vi "scrollToZoom.vi"(8 "stop":refnum<vi>, 9 "Don't need to press Ctrl To ZoomIn/ZoomOut":bool, 10 "ROI數量":i32=1, 11 "VI in":refnum<vi>) -> ()   [LabVIEW 2015]
panel:
  in  "stop":bool
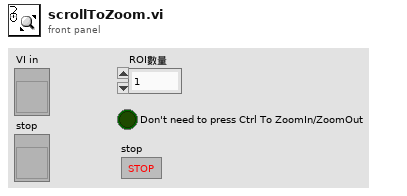
[diagram p1: front panel]
types:
  T1 = cluster{"ImageDataArray":cluster{"ImageName":string, "ImageZoom":dbl}, refnum<vi>}[]
  T2 = cluster{cluster{"Label.Text":string, dbl}, refnum<vi>}
  T3 = enum16{"Always On", "Always Off", "Off While Running"}
  T4 = cluster{"Global Rectangle":i32[], "Contours":cluster{"Contour Type":u32, "ROI Type":u32, "Points":i32[]}[]}
  T5 = typedef "ROI Descriptor" = cluster{"Global Rectangle":i32[], "Contours":cluster{"ID":enum32{"External", "Internal"}, "Type":u32, "Coordinates":i32[]}[]}
  T6 = cluster{"ID":enum32{"External", "Internal"}, "Type":u32, "Coordinates":i32[]}[]
  T7 = cluster{"ID":enum32{"External", "Internal"}, "Type":u32, "Coordinates":i32[]}
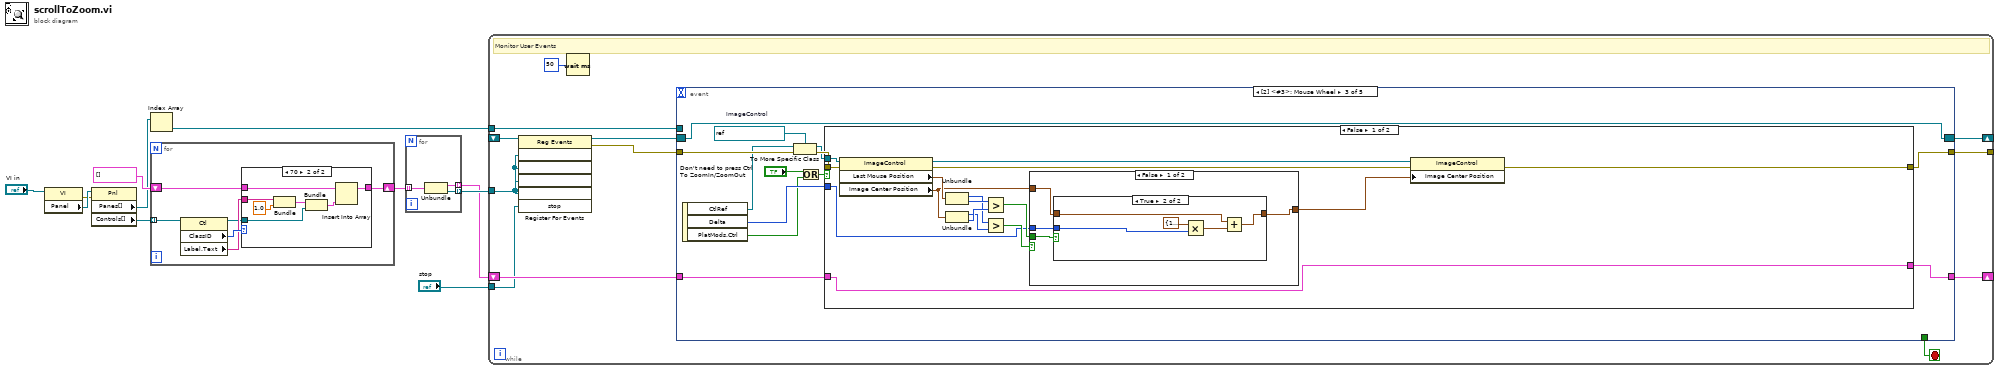
[diagram p0: block diagram]
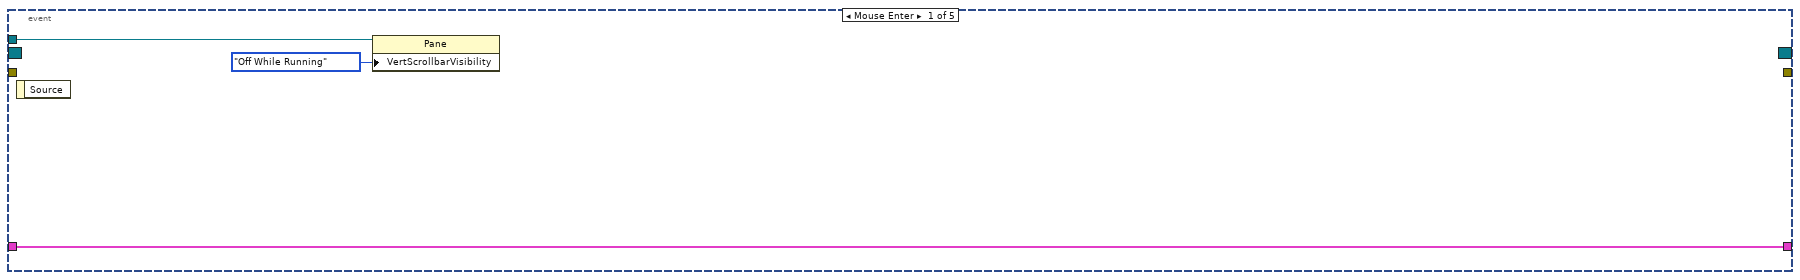
[diagram p3: hidden frame]
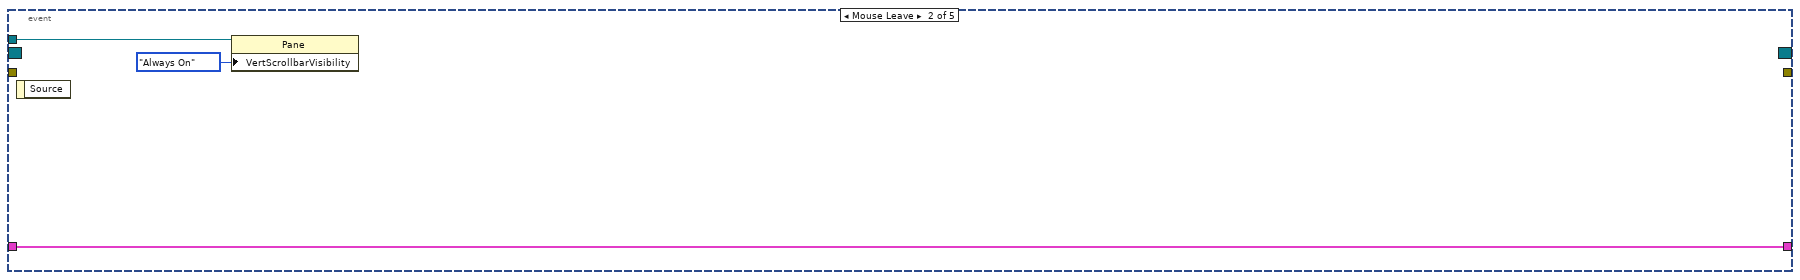
[diagram p4: hidden frame]
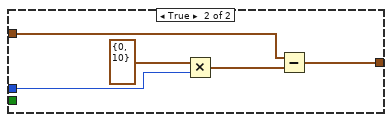
[diagram p6: hidden frame]
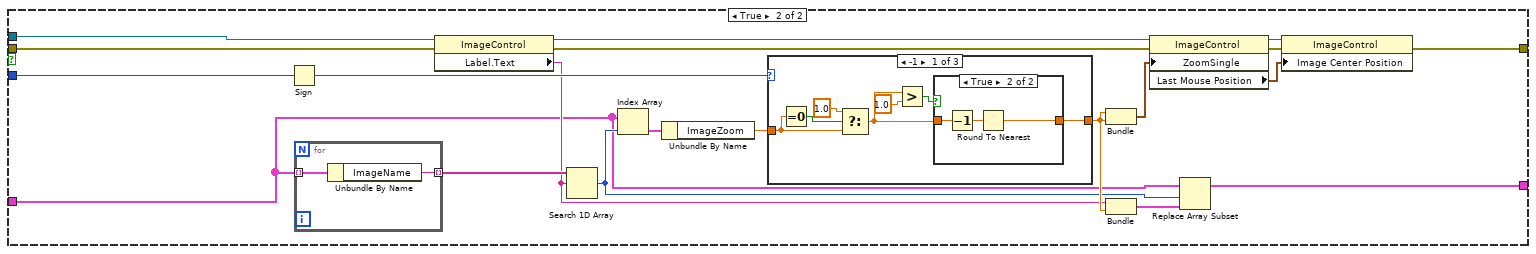
[diagram p7: hidden frame]
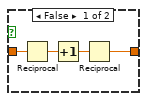
[diagram p8: hidden frame]
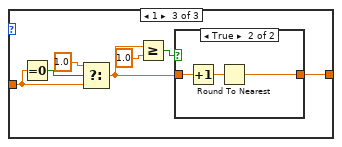
[diagram p10: hidden frame]
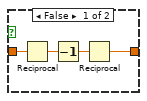
[diagram p11: hidden frame]
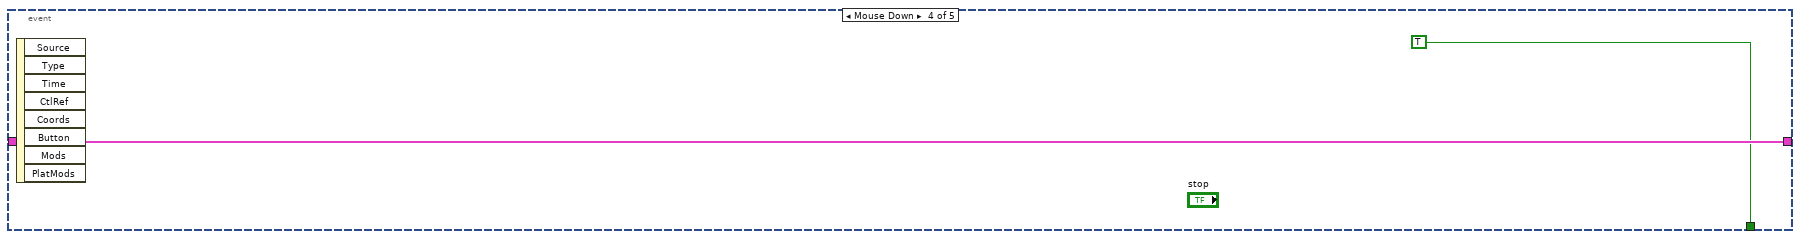
[diagram p12: hidden frame]
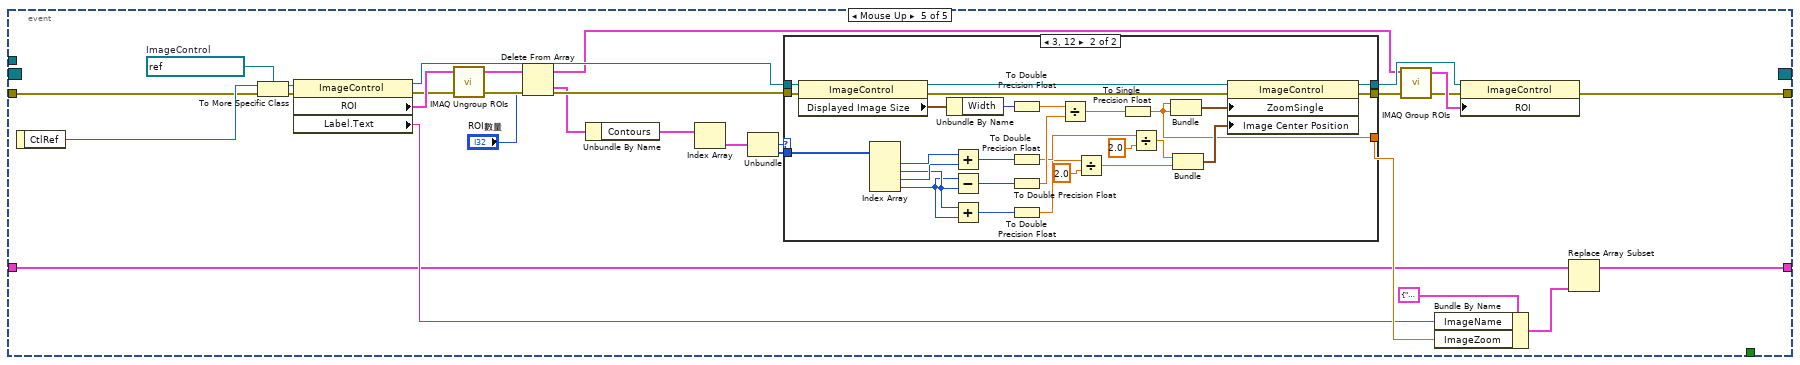
[diagram p13: hidden frame]
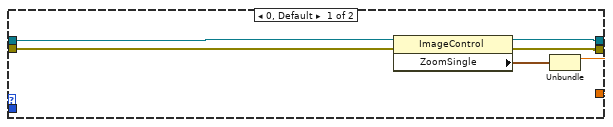
[diagram p14: hidden frame]
diagram:
  n1 = property class="VI"(reference="VI in") -> (error out=w7:errorcluster, "Panel"=w8:refnum<vi>)  [unwired: 1 in, 1 out]
  n2 = property class="Pnl"(reference=w8, error in=w7) -> ("Panes[]"=w9:refnum<vi>[], "Controls[]"=w6:refnum<vi>[])  [unwired: 2 out]
  n3 = Index Array(array=w9) -> (element=w5:refnum<vi>)  [unwired: 1 in]
  n4 = for {
    shift-right: [w15] -> w3
    shift-left: T1 [] -> [w16]
    tunnel: w6 -> [w12] mode=indexing
    n5 = property class="Ctl"(reference=w12) -> (reference out=w13:refnum<vi>, "ClassID"=w17:u32, "Label.Text"=w14:string)  [unwired: 1 in, 1 out]
    n6 = case shown="70" w17 {
      tunnel: w16 -> [w18 w21]
      tunnel: [w18 w19] -> w15
      tunnel: w14 -> [_ w24]
      tunnel: w13 -> [_ w22]
      frame 0, Default {
      }
      frame 70 {
        n7 = Bundle("Label.Text"=w24, 1.0) -> (w23:cluster{"Label.Text":string, dbl})  [unwired: 1 in]
        n8 = Bundle(w23, w22) -> (w20:T2)  [unwired: 1 in]
        n9 = Insert Into Array(array=w21, new element=w20) -> (w19:T1)  [unwired: 1 in]
      }
    }
  }
  n10 = for {
    tunnel: w3 -> [w28] mode=indexing
    tunnel: [w26] -> w4 mode=indexing
    tunnel: [w27] -> w2 mode=indexing
    n11 = Unbundle(w28) -> ("ImageDataArray"=w27:cluster{"ImageName":string, "ImageZoom":dbl}, w26:refnum<vi>)
  }
  n12 = while {
    tunnel: [w38] -> _
    tunnel: w5 -> [w37]
    shift-right: [w36] -> _
    shift-left: _ -> [w29]
    tunnel: w4 -> [w34]
    shift-right: [w32] -> _
    shift-left: w2 -> [w33]
    tunnel: "stop" -> [w30]
    stop <- w31 stop-if-true
    # "Monitor User Events"
    n13 = register-events(reference=w29, w34, w34, w34, w34, w30) -> (reference out=w40:refnum<event-registration>, error out=w39:errorcluster)  [unwired: 1 in]
    n14 = Wait (ms)(milliseconds to wait=u32 50) -> ()  [unwired: 1 out]
    n15 = event shown="[2] <#3>: Mouse Wheel" {
      selector: w40 -> [_ _ w58 _ _]
      dyn-events: [_ _ w58 _ _] -> w36
      timeout: _ -> [_ _ _ _ _]
      tunnel: w39 -> [_ _ w56 _ w162]
      tunnel: [_ _ w57 _ w163] -> w38
      tunnel: w37 -> [w42 w45 _ _ _]
      tunnel: w33 -> [w41 w44 w48 w143 w145]
      tunnel: [w41 w44 w47 w143 w144] -> w32
      tunnel: [_ _ _ TRUE _] -> w31
      event Mouse Enter {
        n16 = event-data() -> ()  [unwired: 1 in, 1 out]
        n17 = property class="Pane"(reference=w42, "VertScrollbarVisibility"=T3."Off While Running" ("Vertical Scrollbar Visibility")) -> ()  [unwired: 1 in, 2 out]
      }
      event Mouse Leave {
        n18 = event-data() -> ()  [unwired: 1 in, 1 out]
        n19 = property class="Pane"(reference=w45, "VertScrollbarVisibility"=T3."Always On" ("Vertical Scrollbar Visibility")) -> ()  [unwired: 1 in, 2 out]
      }
      event Mouse Wheel {
        w59 = refnum<vi> refnum  # ImageControl
        n20 = event-data() -> ("CtlRef"=w55:refnum<vi>, "Delta"=w50:i32, "PlatMods.Ctrl"=w49:bool)  [unwired: 1 in]
        n21 = To More Specific Class(target class=w59, reference=w55, error in=w56) -> (specific class reference=w53:refnum<vi>, error out=w54:errorcluster)
        n22 = Or(x="Don't need to press Ctrl To ZoomIn/ZoomOut", y=w49) -> (x .or. y?=w51:bool)
        n23 = case shown="False" w51 {
          tunnel: [w64 w105] -> w57
          tunnel: w50 -> [w62 w104]
          tunnel: w54 -> [w65 w103]
          tunnel: w53 -> [w68 w100]
          tunnel: w48 -> [w60 w92]
          tunnel: [w60 w91] -> w47
          frame False {
            n24 = property class="ImageControl"(reference=w68, error in=w65) -> (reference out=w67:refnum<vi>, error out=w66:errorcluster, "Last Mouse Position"=w73:cluster{"X":i32, "Y":i32}, "Image Center Position"=w63:cluster{"X":u32, "Y":u32})
            n25 = Unbundle(w73) -> ("X"=w72:i32, "Y"=w75:i32)
            n26 = Unbundle(w63) -> ("X"=w71:u32, "Y"=w74:u32)
            n27 = Greater?(x=w75, y=w74) -> (0:w69:bool)
            n28 = Greater?(x=w72, y=w71) -> (0:w70:bool)
            n29 = case shown="False" w70 {
              tunnel: w69 -> [w79 _]
              tunnel: w63 -> [w78 w90]
              tunnel: w62 -> [w77 w88]
              tunnel: [w76 w86] -> w61
              frame False {
                n30 = case shown="True" w79 {
                  tunnel: w78 -> [w80 w83]
                  tunnel: w77 -> [_ w82]
                  tunnel: [w80 w81] -> w76
                  frame False {
                  }
                  frame True {
                    n31 = Multiply(x=cluster{"X":u32, "Y":u32} {"X"=10, "Y"=0} ("y"), y=w82) -> (x*y=w84:cluster{"X":u32, "Y":u32})
                    n32 = Add(x=w83, y=w84) -> (x+y=w81:cluster{"X":u32, "Y":u32})
                  }
                }
              }
              frame True {
                n33 = Multiply(x=cluster{"X":u32, "Y":u32} {"X"=0, "Y"=10} ("y"), y=w88) -> (x*y=w87:cluster{"X":u32, "Y":u32})
                n34 = Subtract(x=w90, y=w87) -> (x-y=w86:cluster{"X":u32, "Y":u32})
              }
            }
            n35 = property class="ImageControl"(reference=w67, error in=w66, "Image Center Position"=w61) -> (error out=w64:errorcluster)  [unwired: 1 out]
          }
          frame True {
            n36 = Sign(1:w104) -> (0:w110:i32)
            n37 = for {
              tunnel: w92 -> [w112] mode=indexing
              tunnel: [w111] -> w97 mode=indexing
              n38 = Unbundle By Name(w112) -> ("ImageName"=w111:string)
            }
            n39 = property class="ImageControl"(reference=w100, error in=w103) -> (reference out=w101:refnum<vi>, error out=w102:errorcluster, "Label.Text"=w96:string)
            n40 = Search 1D Array(1D array=w97, element=w96) -> (index of element=w93:i32)  [unwired: 1 in]
            n41 = Index Array(array=w92, index=w93) -> (element=w95:cluster{"ImageName":string, "ImageZoom":dbl})
            n42 = Unbundle By Name(w95) -> ("ImageZoom"=w94:dbl)
            n43 = case shown="-1" w110 {
              tunnel: [w117 w127 w132] -> w98
              tunnel: w94 -> [w113 w127 w129]
              frame -1 {
                n44 = Equal To 0?(x=w113) -> (x = 0?=w116:bool)
                n45 = Select(t=1.0 ("y"), s=w116, f=w113) -> (s? t:f=w114:dbl)
                n46 = Greater?(x=w114, y=1.0) -> (0:w118:bool)
                n47 = case shown="True" w118 {
                  tunnel: [w121 w125] -> w117
                  tunnel: w114 -> [w120 w124]
                  frame False {
                    n48 = Reciprocal(x=w120) -> (1/x=w122:dbl)
                    n49 = Increment(x=w122) -> (x+1=w123:dbl)
                    n50 = Reciprocal(x=w123) -> (1/x=w121:dbl)
                  }
                  frame True {
                    n51 = Decrement(x=w124) -> (x-1=w126:dbl)
                    n52 = Round To Nearest(number=w126) -> (nearest integer value=w125:dbl)
                  }
                }
              }
              frame 0, Default {
              }
              frame 1 {
                n53 = Equal To 0?(x=w129) -> (x = 0?=w131:bool)
                n54 = Select(t=1.0 ("y"), s=w131, f=w129) -> (s? t:f=w128:dbl)
                n55 = Greater Or Equal?(x=w128, y=1.0) -> (x >= y?=w133:bool)
                n56 = case shown="True" w133 {
                  tunnel: [w136 w140] -> w132
                  tunnel: w128 -> [w135 w139]
                  frame False {
                    n57 = Reciprocal(x=w135) -> (1/x=w137:dbl)
                    n58 = Decrement(x=w137) -> (x-1=w138:dbl)
                    n59 = Reciprocal(x=w138) -> (1/x=w136:dbl)
                  }
                  frame True {
                    n60 = Increment(x=w139) -> (x+1=w141:dbl)
                    n61 = Round To Nearest(number=w141) -> (nearest integer value=w140:dbl)
                  }
                }
              }
            }
            n62 = Bundle("ImageZoom"=w98, "ImageZoom"=w98) -> (w109:cluster{"ImageZoom":dbl, "ImageZoom":dbl})  [unwired: 1 in]
            n63 = Bundle("Label.Text"=w96, "ImageZoom"=w98) -> (w99:cluster{"Label.Text":string, "ImageZoom":dbl})  [unwired: 1 in]
            n64 = property class="ImageControl"(reference=w101, error in=w102, "ZoomSingle"=w109) -> (reference out=w107:refnum<vi>, error out=w106:errorcluster, "Last Mouse Position"=w108:cluster{"X":i32, "Y":i32})
            n65 = Replace Array Subset(array=w92, new element=w99, index=w93) -> (w91:cluster{"ImageName":string, "ImageZoom":dbl}[])
            n66 = property class="ImageControl"(reference=w107, error in=w106, "Image Center Position"=w108) -> (error out=w105:errorcluster)  [unwired: 1 out]
          }
        }
      }
      event Mouse Down {
        n67 = event-data() -> ()  [unwired: 1 in, 8 out]
      }
      event Mouse Up {
        w165 = refnum<vi> refnum  # ImageControl
        n68 = event-data() -> ("CtlRef"=w166:refnum<vi>)  [unwired: 1 in]
        n69 = To More Specific Class(target class=w165, reference=w166, error in=w162) -> (specific class reference=w164:refnum<vi>, error out=w161:errorcluster)
        n70 = property class="ImageControl"(reference=w164, error in=w161) -> (reference out=w160:refnum<vi>, error out=w157:errorcluster, "ROI"=w158:T4, "Label.Text"=w159:string)
        n71 = call "IMAQ Ungroup ROIs"("error in (no error)"=w157, "ROI Descriptor"=w158) -> ("error out"=w156:errorcluster, "ROI Descriptors out"=w152:T5[])  [unwired: 2 in]
        n72 = Delete From Array(array=w152, index="ROI數量") -> (deleted portion=w148:T5, array with subset deleted=w150:T5[])  [unwired: 1 in]
        n73 = Unbundle By Name(w148) -> ("Contours"=w171:T6)
        n74 = Index Array(array=w171) -> (element=w155:T7)  [unwired: 1 in]
        n75 = Unbundle(w155) -> ("Type"=w154:u32, "Coordinates"=w153:i32[])  [unwired: 1 out]
        n76 = case shown="3, 12" w154 {
          tunnel: w153 -> [_ w178]
          tunnel: w160 -> [w177 w205]
          tunnel: [w176 w185] -> w170
          tunnel: w156 -> [w174 w184]
          tunnel: [w173 w182] -> w147
          tunnel: [w172 w179] -> w167
          frame 0, Default {
            n77 = property class="ImageControl"(reference=w177, error in=w174) -> (reference out=w176:refnum<vi>, error out=w173:errorcluster, "ZoomSingle"=w175:cluster{"X":sgl, "Y":sgl})
            n78 = Unbundle(w175) -> ("X"=w172:sgl)  [unwired: 1 out]
          }
          frame 3, 12 {
            n79 = property class="ImageControl"(reference=w205, error in=w184) -> (reference out=w186:refnum<vi>, error out=w183:errorcluster, "Displayed Image Size"=w204:cluster{"Width":u32, "Height":u32})
            n80 = Index Array(array=w178) -> (element #1=w203:i32, element #2=w200:i32, element #3=w202:i32, element #4=w199:i32)  [unwired: 4 in]
            n81 = Unbundle By Name(w204) -> ("Width"=w194:u32)
            n82 = Add(x=w203, y=w202) -> (x+y=w191:i32)
            n83 = Subtract(x=w199, y=w200) -> (x-y=w196:i32)
            n84 = Add(x=w200, y=w199) -> (x+y=w189:i32)
            n85 = To Double Precision Float(number=w194) -> (double precision float=w193:dbl)
            n86 = To Double Precision Float(number=w191) -> (double precision float=w190:dbl)
            n87 = To Double Precision Float(number=w196) -> (double precision float=w195:dbl)
            n88 = To Double Precision Float(number=w189) -> (double precision float=w188:dbl)
            n89 = Divide(x=w193, y=w195) -> (x/y=w197:dbl)
            n90 = Divide(x=w188, y=2.0) -> (x/y=w180:dbl)
            n91 = To Single Precision Float(number=w197) -> (single precision float=w179:sgl)
            n92 = Divide(x=w190, y=2.0) -> (x/y=w181:dbl)
            n93 = Bundle(w179, w179) -> (w198:cluster{sgl, sgl})  [unwired: 1 in]
            n94 = Bundle(w181, w180) -> (w187:cluster{dbl, dbl})  [unwired: 1 in]
            n95 = property class="ImageControl"(reference=w186, error in=w183, "ZoomSingle"=w198, "Image Center Position"=w187) -> (reference out=w185:refnum<vi>, error out=w182:errorcluster)
          }
        }
        n96 = call "IMAQ Group ROIs"("error in (no error)"=w147, "ROI Descriptors"=w150) -> ("error out"=w146:errorcluster, "ROI Descriptor out"=w149:T5)  [unwired: 2 in]
        n97 = Bundle By Name(cluster=cluster{"ImageName":string, "ImageZoom":dbl} {"ImageName"="", "ImageZoom"=0.0}, "ImageName"=w159, "ImageZoom"=w167) -> (w168:cluster{"ImageName":string, "ImageZoom":dbl})
        n98 = property class="ImageControl"(reference=w170, error in=w146, "ROI"=w149) -> (error out=w163:errorcluster)  [unwired: 1 out]
        n99 = Replace Array Subset(array=w145, new element=w168) -> (w144:cluster{"ImageName":string, "ImageZoom":dbl}[])  [unwired: 1 in]
      }
    }
  }
